vi "Write Data.vi"(0 "reference in":refnum<class "RPC.lvclass">, 5 "error in (no error)":errorcluster) -> (14 "reference out":refnum<class "RPC.lvclass">, 19 "error out":errorcluster)   [LabVIEW 2022 SP3, in "RPC.lvclass"]
uses:
  RPC.lvclass
  API/GSwFormDSP_class/GSwFormDSP.lvclass
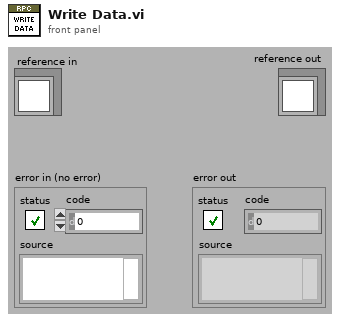
[diagram p1: front panel]
types:
  T1 = enum16{"big-endian, network order", "native, host order", "little-endian"}
  T2 = typedef "RPC.lvclass/ObjectAttributes.ctl" = cluster{"File Refnum":refnum<file>, "File total size":i32, "Offset from start of file":i32, "Time Type":enum16{"Response", "Drive"}, "Full Scale":dbl[unit], "New Time Data Obj?":bool, "Header":cluster{"Num Header":i32, "Num Parameter":i32, "Nb Channels":i32, "dT":dbl, "Number of Groups":i32, "Group size":i32, "Units":string[], "Names":string[], "Sensitivity":dbl[], "Complete header":string[]}, "Time Data":refnum<class "GSwFormDSP.lvclass">}
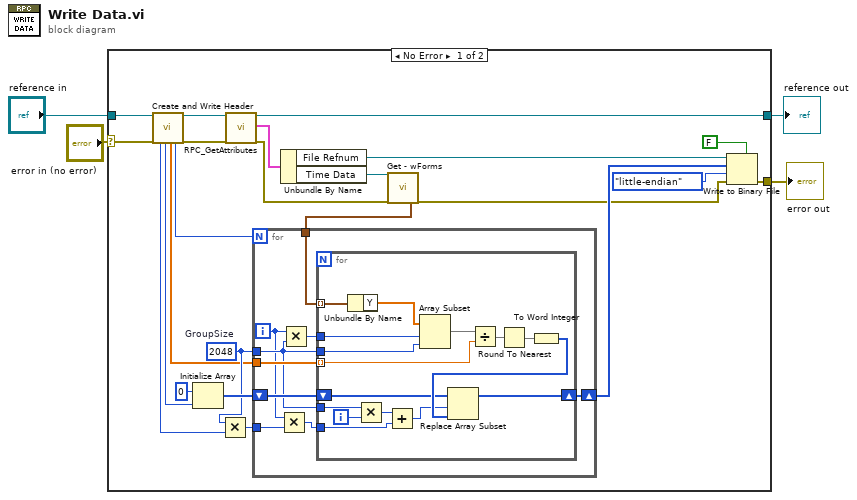
[diagram p0: block diagram]
diagram:
  n1 = case shown="No Error" "error in (no error)" {
    selector: "error in (no error)" -> [w23 w54]
    tunnel: [w6 w54] -> w3
    tunnel: [w27 w53] -> w1
    tunnel: "reference in" -> [w25 w53]
    frame No Error {
      w16 = 2048  # GroupSize
      n2 = call "Create and Write Header.vi"("reference in"=w25, "error in (no error)"=w23) -> ("Nb Channels"=w11:i32, "Total Nb Samples"=w12:i32, "Scaling factors"=w13:dbl[], "Nb Groups"=w14:i32, "reference out"=w24:refnum<class "RPC.lvclass">, "error out"=w22:errorcluster)  [unwired: 12 in]
      n3 = Initialize Array(i16 0 ("element"), w12) -> (w18:i16[])
      n4 = Multiply(x=w16, y=w11) -> (x*y=w15:i32)
      n5 = call "RPC_GetAttributes.vi"("reference in"=w24, "error in (no error)"=w22) -> ("reference out"=w27:refnum<class "RPC.lvclass">, "attributes"=w26:T2, "error out"=w8:errorcluster)  [unwired: 14 in, 1 out]
      n6 = Unbundle By Name(w26) -> ("File Refnum"=w10:refnum<file>, "Time Data"=w9:refnum<class "GSwFormDSP.lvclass">)
      n7 = call-dynamic "Get - wForms.vi"("reference in"=w9, "error in (no error)"=w8) -> ("wForms"=w5:waveform(dbl)[], "error out"=w7:errorcluster)  [unwired: 14 in, 2 out]
      n8 = for {
        N: w14 -> [_]
        shift-right: [w34] -> w17
        shift-left: w18 -> [w36]
        tunnel: w13 -> [w33]
        tunnel: w16 -> [w32]
        tunnel: w15 -> [w31]
        tunnel: w5 -> [w28]
        i -> [w30]
        n9 = Multiply(x=w30, y=w31) -> (x*y=w29:i32)
        n10 = Multiply(x=w30, y=w32) -> (x*y=w35:i32)
        n11 = for {
          shift-right: [w47] -> w34
          shift-left: w36 -> [w48]
          tunnel: w35 -> [w43]
          tunnel: w33 -> [w46] mode=indexing
          tunnel: w32 -> [w45]
          tunnel: w32 -> [w41]
          tunnel: w29 -> [w39]
          tunnel: w28 -> [w38] mode=indexing
          i -> [w42]
          n12 = Unbundle By Name(w38) -> ("Y"=w37:dbl[])
          n13 = Multiply(x=w41, y=w42) -> (x*y=w40:i32)
          n14 = Add(x=w40, y=w39) -> (x+y=w44:i32)
          n15 = Array Subset(array=w37, index=w43, length=w45) -> (w52:dbl[])
          n16 = Divide(x=w52, y=w46) -> (x/y=w51:dbl[])
          n17 = Round To Nearest(number=w51) -> (nearest integer value=w50:dbl[])
          n18 = To Word Integer(number=w50) -> (16bit integer=w49:i16[])
          n19 = Replace Array Subset(array=w48, new element=w49, index=w44) -> (w47:i16[])
        }
      }
      n20 = Write to Binary File(file (use dialog)=w10, data=w17, error in=w7, 5:FALSE ("prepend array or string size? (T)"), 9:T1."little-endian" ("byte order (0:big-endian, network order)")) -> (error out=w6:errorcluster)  [unwired: 3 out]
    }
    frame Error {
    }
  }
  "error out" <- w3
  "reference out" <- w1
